vi "Ranked Peak Finder.vi"(4 "waveform":waveform(dbl)) -> (1 "Peak Coordinates":cluster{"y":dbl, "x":dbl}[](array[cluster]))   [LabVIEW 2013]
uses:
  <vilib>/Analysis/NI_AALPro.lvlib
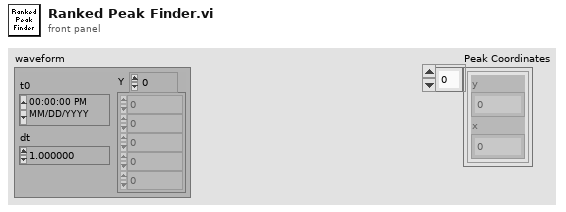
[diagram p1: front panel]
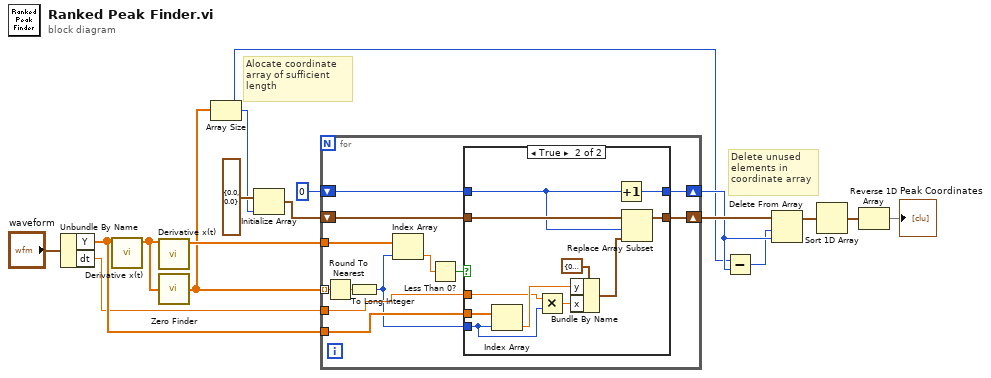
[diagram p0: block diagram]
diagram:
  # "Alocate coordinate\narray of sufficient\nlength"
  # "Delete unused\nelements in\ncoordinate array"
  n1 = Unbundle By Name("waveform") -> ("Y"=w8:dbl[], "dt"=w5:dbl)
  n2 = call <vilib>:"Derivative x(t).vi"("X"=w8) -> ("dX/dt"=w16:dbl[])  [unwired: 9 in, 1 out]
  n3 = call <vilib>:"Derivative x(t).vi"("X"=w16) -> ("dX/dt"=w14:dbl[])  [unwired: 9 in, 1 out]
  n4 = call "Zero Finder.vi"("array"=w16) -> ("fractional zeros"=w4:dbl[])  [unwired: 4 in]
  n5 = Array Size(array=w4) -> (size(s)=w6:i32)
  n6 = Initialize Array(cluster{"y":dbl, "x":dbl} {"y"=0.0, "x"=0.0}, w6) -> (w7:cluster{"y":dbl, "x":dbl}[])
  n7 = for {
    tunnel: w14 -> [w21]
    tunnel: w4 -> [w22] mode=indexing
    shift-right: [w27] -> w11
    shift-left: 0 -> [w28]
    shift-right: [w25] -> w12
    shift-left: w7 -> [w26]
    tunnel: w8 -> [w24]
    tunnel: w5 -> [w23]
    n8 = Round To Nearest(number=w22) -> (nearest integer value=w18:dbl)
    n9 = To Long Integer(number=w18) -> (32bit integer=w17:i32)
    n10 = Index Array(array=w21, index=w17) -> (element=w20:dbl)
    n11 = Less Than 0?(x=w20) -> (x < 0?=w19:bool)
    n12 = case shown="True" w19 {
      tunnel: w28 -> [w30 w36]
      tunnel: [w30 w41] -> w27
      tunnel: w26 -> [w29 w40]
      tunnel: w17 -> [_ w32]
      tunnel: [w29 w39] -> w25
      tunnel: w24 -> [_ w38]
      tunnel: w23 -> [_ w31]
      frame False {
      }
      frame True {
        n13 = Index Array(array=w38, index=w32) -> (element=w34:dbl)
        n14 = Multiply(x=w31, y=w32) -> (x*y=w33:dbl)
        n15 = Bundle By Name(cluster=cluster{"y":dbl, "x":dbl} {"y"=0.0, "x"=0.0}, "y"=w34, "x"=w33) -> (w35:cluster{"y":dbl, "x":dbl})
        n16 = Increment(x=w36) -> (x+1=w41:i32)
        n17 = Replace Array Subset(array=w40, new element=w35, index=w36) -> (w39:cluster{"y":dbl, "x":dbl}[])
      }
    }
  }
  n18 = Subtract(x=w6, y=w11) -> (x-y=w10:i32)
  n19 = Delete From Array(array=w12, length=w10, index=w11) -> (array with subset deleted=w3:cluster{"y":dbl, "x":dbl}[])  [unwired: 1 out]
  n20 = Sort 1D Array(array=w3) -> (sorted array=w2:cluster{"y":dbl, "x":dbl}[])
  n21 = Reverse 1D Array(array=w2) -> (reversed array=→"Peak Coordinates":cluster{"y":dbl, "x":dbl}[])
